vi "SendShutdownCommand.vi"(10 "dummy input":variant, 11 "Source VI":string) -> ()   [LabVIEW 2017, in "GFG library.lvlib"]
doc: "SciScan 1.2 160622\nThis VI sets the variable \"Shutdown\" to TRUE and thereby sends a shutdown event to all listeners. Wire any data type to the dummy input to establish dataflow timing."
uses:
  GFG/GFG library.lvlib
  GFG/GFGfpRefGet.vi
panel:
  out "error out":errorcluster
  in  "error in (no error)":errorcluster
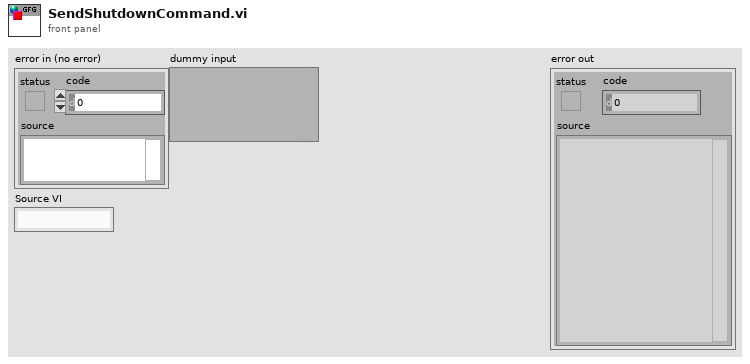
[diagram p1: front panel]
types:
  T1 = cluster{"WaveformChartRef":refnum<vi>, "DigitalRef":refnum<vi>, "ArrayRef":refnum<vi>, "TabControlRef":refnum<vi>, "EnumRef":refnum<vi>, "RingRef":refnum<vi>, "BooleanRef":refnum<vi>, "KnobRef":refnum<vi>, "SlideRef":refnum<vi>, "PathRef":refnum<vi>, "StringRef":refnum<vi>, "ComboBox":refnum<vi>, "WaveformGraphRef":refnum<vi>}
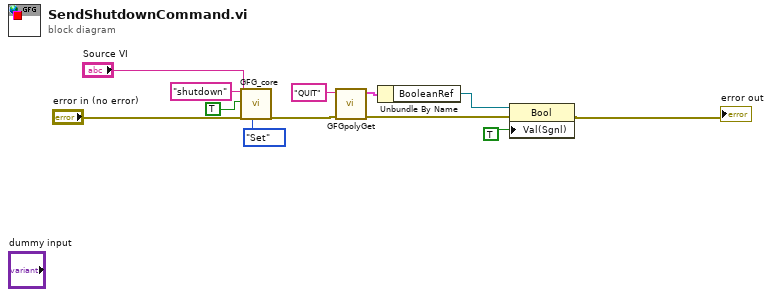
[diagram p0: block diagram]
diagram:
  n1 = call "GFG_core.vi"("Variable Name in"="shutdown", "Variant in"=TRUE, "Source VI"="Source VI", "error in (no error)"="error in (no error)", "Action"=enum16{"Init", "Set", "Get"}."Set") -> ("error out"=w6:errorcluster)  [unwired: 8 in, 6 out]
  n2 = call-poly "GFGpolyGet.vi"("error in (no error)"=w6, "Variable Name in"="QUIT") -> ("error out"=w2:errorcluster, "output cluster"=w5:T1)  [unwired: 8 in]
  n3 = Unbundle By Name(w5) -> ("BooleanRef"=w4:refnum<vi>)
  n4 = property class="Bool"(reference=w4, error in=w2, "Val(Sgnl)"=TRUE) -> (error out=→"error out":errorcluster)  [unwired: 1 out]
